vi "U8 Array Conversion.vi"(6 "Reverse":bool, 7 "Conversion Type":T1, 11 "U8 Array":u8[](array[numeric]) format="%02x") -> (3 "Conversion Output":variant)   [LabVIEW 2025]
uses:
  Conversion Type.ctl
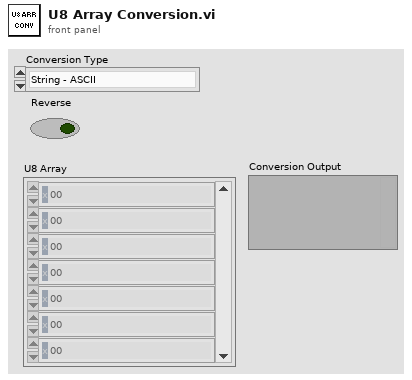
[diagram p1: front panel]
types:
  T1 = typedef "Conversion Type.ctl" = enum16{"String - ASCII", "String - HEX", "Numeric - DEC"}
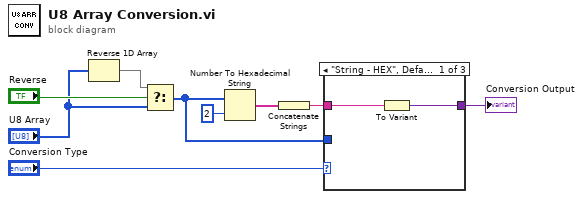
[diagram p0: block diagram]
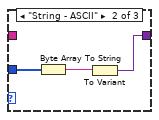
[diagram p2: hidden frame]
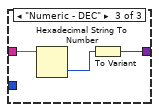
[diagram p3: hidden frame]
diagram:
  n1 = Reverse 1D Array(array="U8 Array") -> (reversed array=w8:u8[])
  n2 = Select(t=w8, s="Reverse", f="U8 Array") -> (s? t:f=w2:u8[])
  n3 = Number To Hexadecimal String(1:i16 2 ("width (-)"), 2:w2) -> (0:w6:string[])
  n4 = Concatenate Strings(w6) -> (w5:string)
  n5 = case shown="\"String - HEX\", Default" "Conversion Type" {
    tunnel: w5 -> [w11 _ w17]
    tunnel: [w10 w14 w15] -> w3
    tunnel: w2 -> [_ w12 _]
    frame "String - HEX", Default {
      n6 = To Variant(anything=w11) -> (Variant=w10:variant)
    }
    frame "String - ASCII" {
      n7 = Byte Array To String(unsigned byte array=w12) -> (string=w13:string)
      n8 = To Variant(anything=w13) -> (Variant=w14:variant)
    }
    frame "Numeric - DEC" {
      n9 = Hexadecimal String To Number(string=w17) -> (number=w16:u32)  [unwired: 2 in, 1 out]
      n10 = To Variant(anything=w16) -> (Variant=w15:variant)
    }
  }
  "Conversion Output" <- w3
